vi "Write Log Summary Dialog.vi"(7 "Console Log in":refnum<class "Console Log.lvclass">, 8 "error in":errorcluster, 11 "Gluing Procedure in":refnum<class "Gluing Procedure.lvclass">) -> (0 "error out":errorcluster, 1 "Step canceled?":bool, 3 "Gluing Procedure out":refnum<class "Gluing Procedure.lvclass">, 5 "Console Log out":refnum<class "Console Log.lvclass">)   [LabVIEW 2011]
uses:
  Procedure Classes/Gluing Procedure/Gluing Procedure.lvclass
  Application Utilities/Console Log/Console Log.lvclass
  Shared Components/Gantry Class/Gantry Class.lvclass
  Shared Components/Config Manager Class/Config Manager Class.lvclass
panel:
  in  "Database Updated?":enum32{"Radio Selection 1", "Radio Selection 2"}(radio)
  in  "Additional Comments:":string
  in  "Operator Name":string
  in  "Cancel Button":bool
  in  "OK Button":bool
  # "The gluing routine has completed!\n\nPlease fill the fields below to complete the log and press OK."
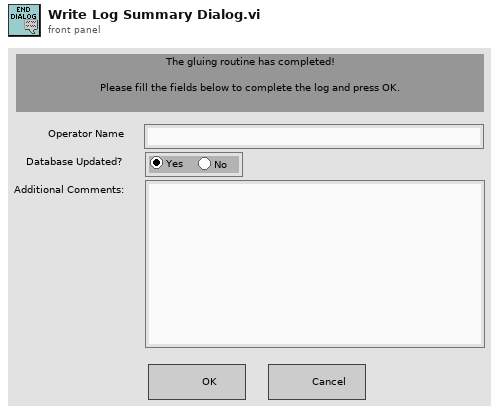
[diagram p1: front panel]
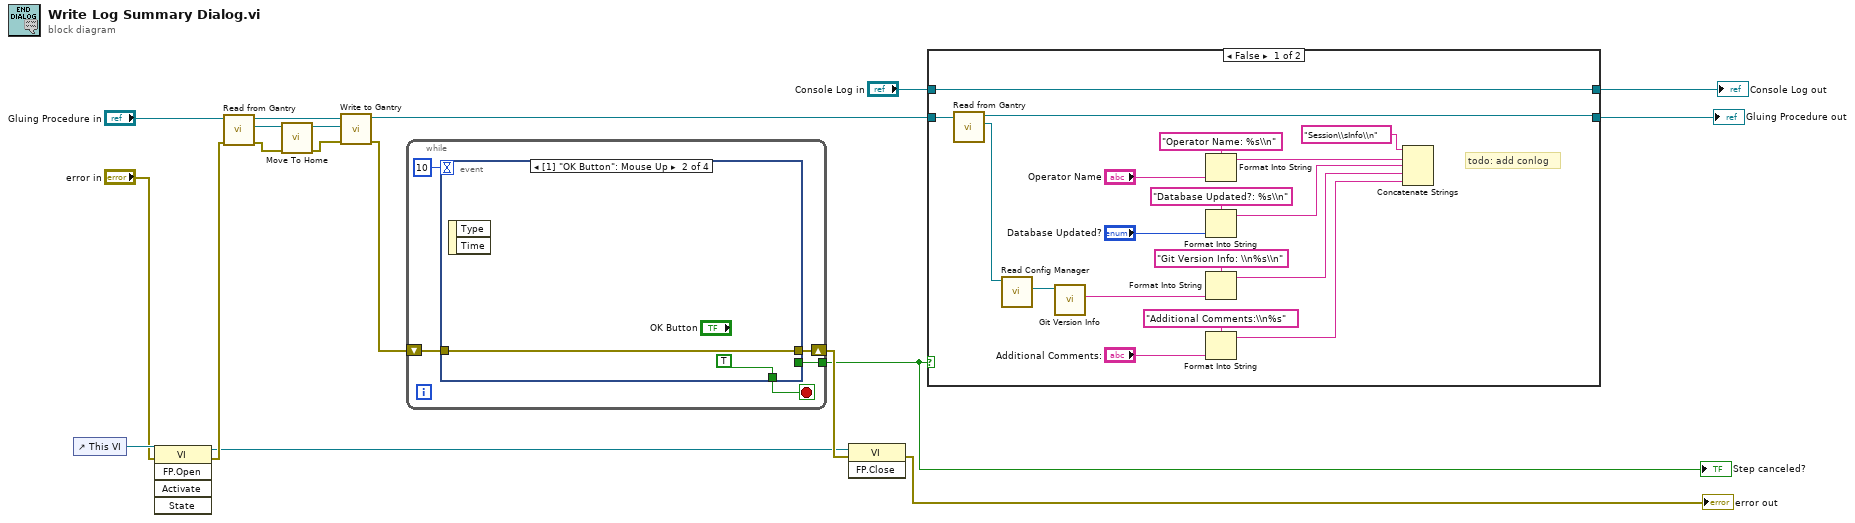
[diagram p0: block diagram]
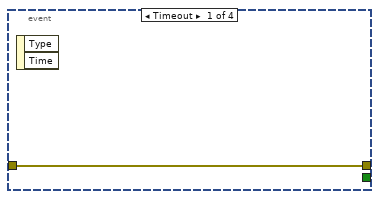
[diagram p3: hidden frame]
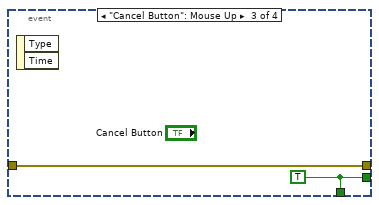
[diagram p4: hidden frame]
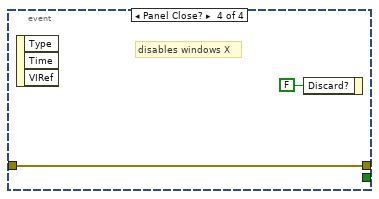
[diagram p5: hidden frame]
diagram:
  n1 = control-ref of="This VI"() -> (w18:refnum<vi>)
  n2 = invoke class="VI" method="FP.Open"(reference=w18, error in="error in") -> (reference out=w7:refnum<vi>, error out=w15:errorcluster)  [unwired: 3 in, 3 out]
  n3 = call "Read from Gantry.vi"("error in (no error)"=w15, "Gluing Procedure in"="Gluing Procedure in") -> ("error out"=w13:errorcluster, "Gantry"=w14:refnum<class "Gantry Class.lvclass">, "Gluing Procedure out"=w12:refnum<class "Gluing Procedure.lvclass">)  [unwired: 7 in]
  n4 = call-dynamic "Move To Home.vi"("error in"=w13, "Gantry in"=w14) -> ("error out"=w10:errorcluster, "Gantry out"=w11:refnum<class "Gantry Class.lvclass">)  [unwired: 8 in]
  n5 = call "Write to Gantry.vi"("error in (no error)"=w10, "Gantry"=w11, "Gluing Procedure in"=w12) -> ("error out"=w9:errorcluster, "Gluing Procedure out"=w3:refnum<class "Gluing Procedure.lvclass">)  [unwired: 7 in]
  n6 = while {
    shift-right: [w21] -> w8
    shift-left: w9 -> [w22]
    tunnel: [w19] -> w6
    stop <- w20 stop-if-true
    n7 = event shown="[1] \"OK Button\": Mouse Up" {
      selector: _ -> [_ _ _ _]
      dyn-events: _ -> [_ _ _ _]
      timeout: 10 -> [_ _ _ _]
      tunnel: w22 -> [w24 w25 w27 w29]
      tunnel: [w24 w25 w27 w29] -> w21
      tunnel: [_ _ w28 _] -> w19
      tunnel: [_ TRUE w28 _] -> w20
      event Timeout {
        n8 = event-data() -> ()  [unwired: 1 in, 2 out]
      }
      event "OK Button": Mouse Up {
        n9 = event-data() -> ()  [unwired: 1 in, 2 out]
      }
      event "Cancel Button": Mouse Up {
        w28 = TRUE
        n10 = event-data() -> ()  [unwired: 1 in, 2 out]
      }
      event Panel Close? {
        # "disables windows X"
        n11 = event-data() -> ()  [unwired: 1 in, 3 out]
        n12 = event-data("Discard?"=FALSE) -> ()  [unwired: 1 in, 1 out]
      }
    }
  }
  "Step canceled?" <- w6
  n13 = invoke class="VI" method="FP.Close"(reference=w7, error in=w8) -> (error out=→"error out":errorcluster)  [unwired: 1 in, 2 out]
  n14 = case shown="False" w6 {
    tunnel: "Console Log in" -> [w48 w50]
    tunnel: [w48 w50] -> w4
    tunnel: w3 -> [w47 w49]
    tunnel: [w31 w49] -> w2
    frame False {
      # "todo: add conlog"
      n15 = call "Read from Gantry.vi"("Gluing Procedure in"=w47) -> ("Gantry"=w46:refnum<class "Gantry Class.lvclass">, "Gluing Procedure out"=w31:refnum<class "Gluing Procedure.lvclass">)  [unwired: 8 in, 1 out]
      n16 = call-dynamic "Read Config Manager.vi"("Gantry in"=w46) -> ("Config Manager"=w45:refnum<class "Config Manager Class.lvclass">)  [unwired: 8 in, 2 out]
      n17 = call "Git Version Info.vi"("Config Manager in"=w45) -> ("Git Data"=w40:string)  [unwired: 8 in, 2 out]
      n18 = Format Into String(format string="Operator Name: %s\\n", "Operator Name") -> (resulting string=w35:string)  [unwired: 2 in, 1 out]
      n19 = Format Into String(format string="Database Updated?: %s\\n", "Database Updated?") -> (resulting string=w34:string)  [unwired: 2 in, 1 out]
      n20 = Format Into String(format string="Git Version Info: \\n%s\\n", w40) -> (resulting string=w33:string)  [unwired: 2 in, 1 out]
      n21 = Format Into String(format string="Additional Comments:\\n%s", "Additional Comments:") -> (resulting string=w32:string)  [unwired: 2 in, 1 out]
      n22 = Concatenate Strings("Session\\sInfo\\n" ("string"), w35, w34, w33, w32) -> ()  [unwired: 1 out]
    }
    frame True {
    }
  }
  "Gluing Procedure out" <- w2
  "Console Log out" <- w4
